vi "calculateDangerOfPosition.vi"(7 "reference":refnum<class "Enemy.lvclass">, 8 "error in (no error)":errorcluster, 9 "Game":refnum<class "Game.lvclass">, 10 "Enemy Robot":refnum<class "Robot.lvclass">, 11 "MarkerSkill in":refnum<class "MarkerSkill.lvclass">) -> (0 "error out":errorcluster, 2 "DangerEnemy":T1[](array[typedef]), 3 "MarkerSkill out":refnum<class "MarkerSkill.lvclass">)   [LabVIEW 2021, in "MarkerSkill.lvclass"]
uses:
  MarkerSkill.lvclass
  Robot_class/Robot.lvclass
  Game_class/Game.lvclass
  Enemy_class/Enemy.lvclass
  dangerEnemy.ctl
  Utilities_class/Utilities.lvclass
  Game_class/Game.lvclass/Game.ctl
  Robot_class/Robot.lvclass/Robot.ctl
  Referee_class/Referee.lvclass/Referee.ctl
  Referee_class/Read enemy_goalie_id.vi
  Robot_class/Read id.vi
  Game_class/Read FieldRef.vi
  Game_class/Read BallRef.vi
  Game_class/Read Referee.vi
  Field_class/Field.lvclass
  Ball_class/Ball.lvclass
  Referee_class/Referee.lvclass
panel:
  in  "weightOfEnemyDistanceToBall":dbl=1.0
  in  "weightOfEnemyDistanceToOurGoal":dbl=1.5
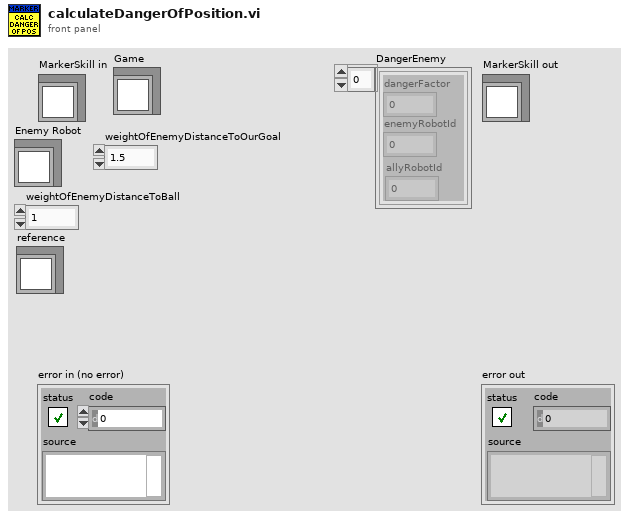
[diagram p1: front panel]
types:
  T1 = typedef "dangerEnemy.ctl" = cluster{"dangerFactor":dbl, "allyRobotId":i32, "enemyRobotId":i32}
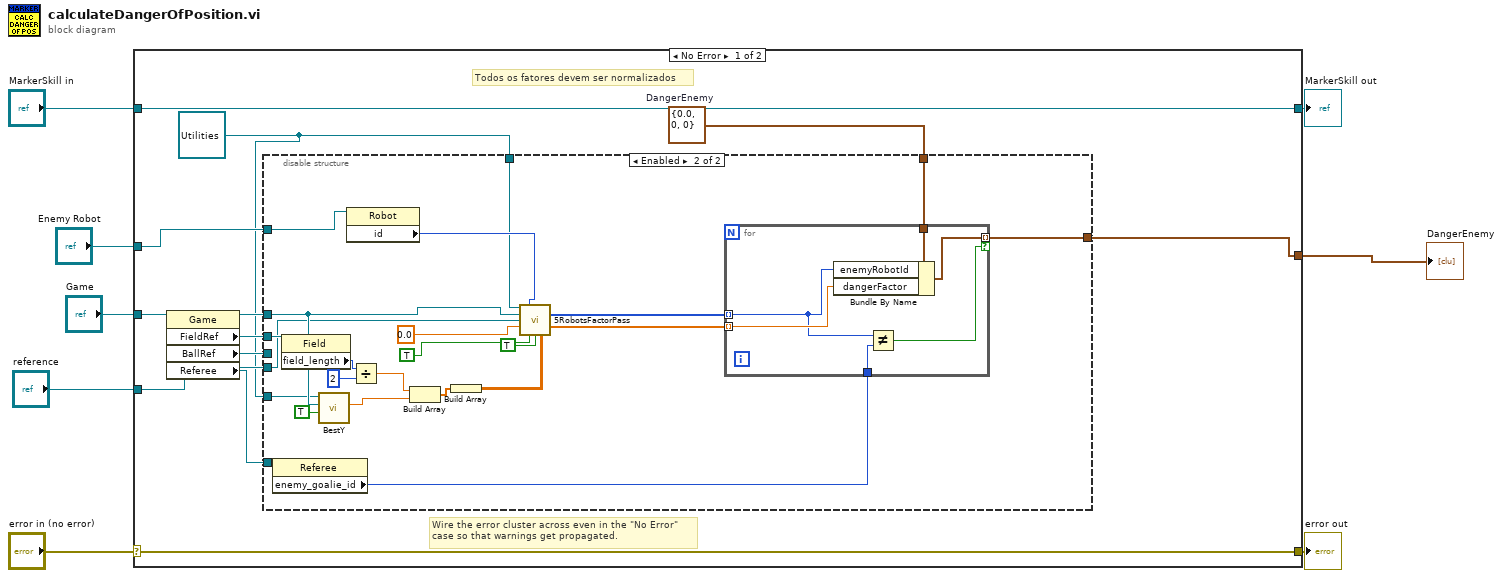
[diagram p0: block diagram]
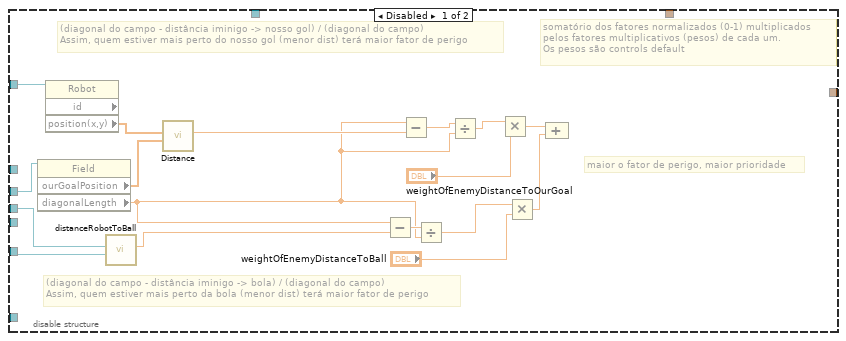
[diagram p2: hidden frame]
diagram:
  n1 = case shown="No Error" "error in (no error)" {
    selector: "error in (no error)" -> [w19 w69]
    tunnel: [w19 w69] -> w7
    tunnel: [w20 w68] -> w5
    tunnel: "MarkerSkill in" -> [w20 w68]
    tunnel: "Enemy Robot" -> [w15 _]
    tunnel: [w11 _] -> w1
    tunnel: "Game" -> [w18 _]
    tunnel: "reference" -> [w13 _]
    frame No Error {
      w10 = refnum<class "Utilities.lvclass"> refnum ("Utilities in")
      w12 = T1 {"dangerFactor"=0.0, "allyRobotId"=0, "enemyRobotId"=0}  # DangerEnemy
      # "Todos os fatores devem ser normalizados"
      # "Wire the error cluster across even in the \"No Error\"\ncase so that warnings get propagated."
      n2 = property class="Game"(reference=w18) -> (reference out=w14:refnum<class "Game.lvclass">, "FieldRef"=w17:refnum<class "Field.lvclass">, "BallRef"=w16:refnum<class "Ball.lvclass">, "Referee"=w9:refnum<class "Referee.lvclass">)  [unwired: 1 in, 1 out]
      n3 = disable-structure shown="Enabled" {
        disable-tunnel: w17 -> [w32 w59]
        disable-tunnel: w16 -> [w31 _]
        disable-tunnel: w15 -> [w30 w61]
        disable-tunnel: w14 -> [_ w52]
        disable-tunnel: w13 -> [_ w51]
        disable-tunnel: w12 -> [_ w47]
        disable-tunnel: [_ w46] -> w11
        disable-tunnel: w10 -> [_ w43]
        disable-tunnel: w10 -> [_ w42]
        disable-tunnel: w9 -> [_ w41]
        frame Disabled {
          # "(diagonal do campo - distância iminigo -> bola) / (diagonal do campo)\nAssim, quem estiver mais perto da bola (menor dist) terá maior fator de perigo"
          # "somatório dos fatores normalizados (0-1) multiplicados\npelos fatores multiplicativos (pesos) de cada um.\nOs pesos são controls default"
          # "maior o fator de perigo, maior prioridade"
          # "(diagonal do campo - distância iminigo -> nosso gol) / (diagonal do campo)\nAssim, quem estiver mais perto do nosso gol (menor dist) terá maior fator de perigo"
          n4 = property class="Field"(reference=w32) -> ("ourGoalPosition"=w38:dbl[], "diagonalLength"=w27:dbl)  [unwired: 1 in, 2 out]
          n5 = property class="Robot"(reference=w30) -> ("id"=w35:i32, "position(x,y)"=w36:dbl[])  [unwired: 1 in, 2 out]
          n6 = call "distanceRobotToBall.vi"("Robot"=w30, "Ball"=w31) -> ("Distance Robot To Ball"=w28:dbl)  [unwired: 7 in, 2 out]
          n7 = call "Distance.vi"("P1"=w38, "P2"=w36) -> ("Distance"=w37:dbl)  [unwired: 7 in, 2 out]
          n8 = Subtract(x=w27, y=w28) -> (x-y=w29:dbl)
          n9 = Subtract(x=w27, y=w37) -> (x-y=w34:dbl)
          n10 = Divide(x=w29, y=w27) -> (x/y=w22:dbl)
          n11 = Divide(x=w34, y=w27) -> (x/y=w26:dbl)
          n12 = Multiply(x=w26, y="weightOfEnemyDistanceToOurGoal") -> (x*y=w25:dbl)
          n13 = Multiply(x=w22, y="weightOfEnemyDistanceToBall") -> (x*y=w24:dbl)
          n14 = Compound Arithmetic op=ADD(w25, w24) -> (w33:dbl)
        }
        frame Enabled {
          n15 = property class="Referee"(reference=w41) -> ("enemy_goalie_id"=w40:i32)  [unwired: 1 in, 2 out]
          n16 = property class="Field"(reference=w59) -> ("field_length"=w58:i32)  [unwired: 1 in, 2 out]
          n17 = call "BestY.vi"("Utilities in"=w42, "Game"=w52, "inimigos"=TRUE) -> ("Best y"=w55:dbl)  [unwired: 2 in, 4 out]
          n18 = property class="Robot"(reference=w61) -> ("id"=w53:i32)  [unwired: 1 in, 2 out]
          n19 = Divide(x=w58, y=2) -> (x/y=w56:dbl)
          n20 = Build Array(w56, w55) -> (w54:dbl[])
          n21 = Build Array(w54) -> (w48:dbl[][])
          n22 = call "5RobotsFactorPass.vi"("Utilities in"=w43, "ID"=w53, "Game in"=w52, "reference"=w51, "Root"=0.0, "Pass?"=TRUE, "Enemy?"=TRUE, "dest_kick"=w48) -> ("Id"=w45:i32[], "FactorPass"=w44:dbl[])  [unwired: 3 in, 3 out]
          n23 = for {
            tunnel: w47 -> [w67]
            tunnel: [w66] -> w46 mode=indexing if=w62
            tunnel: w45 -> [w63] mode=indexing
            tunnel: w44 -> [w65] mode=indexing
            tunnel: w40 -> [w64]
            n24 = Bundle By Name(cluster=w67, "enemyRobotId"=w63, "dangerFactor"=w65) -> (w66:T1)
            n25 = Not Equal?(x=w63, y=w64) -> (x != y?=w62:bool)
          }
        }
      }
    }
    frame Error {
    }
  }
  "error out" <- w7
  "MarkerSkill out" <- w5
  "DangerEnemy" <- w1
